vi "Global Read.vi"(0 "VISA #":string, 3 "error in (no error)":errorcluster) -> (4 "Global for this VISA":T1, 5 "VICI Global Array Out":T2, 6 "Pump Array":string[](array[string]), 7 "Busy":bool, 8 "VISA #":string, 9 "Current Pump":string, 10 "error out":errorcluster)   [LabVIEW 2018, in "VICI M6 M50 Party Mode.lvlib" / "VICI Global Library.lvlib"]
uses:
  VICI Global Library.lvlib
  VICI Global Array.ctl
  VICI Global.ctl
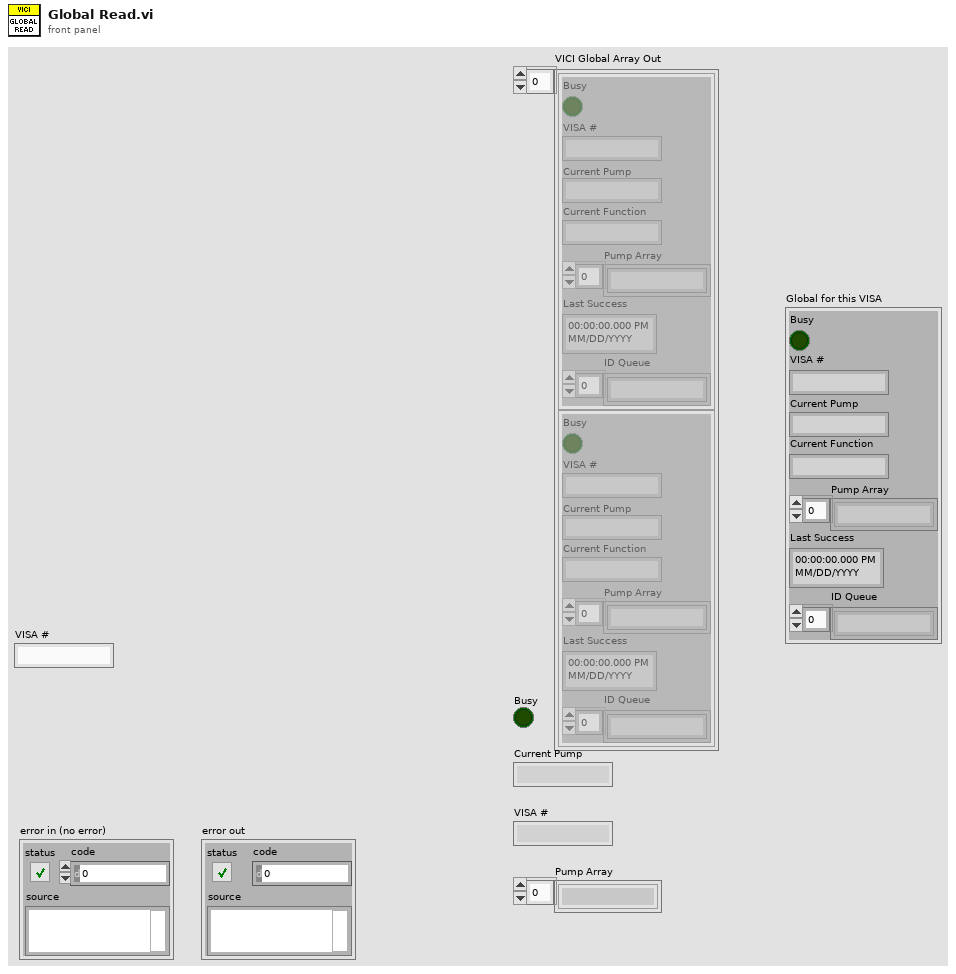
[diagram p1: front panel]
types:
  T1 = typedef "VICI M6 M50 Party Mode.lvlib/VICI Global Library.lvlib/VICI Global.ctl" = cluster{"Busy":bool, "VISA #":string, "Current Pump":string, "Current Function":string, "Pump Array":string[], "Last Success":timestamp, "ID Queue":string[]}
  T2 = typedef "VICI M6 M50 Party Mode.lvlib/VICI Global Library.lvlib/VICI Global Array.ctl" = T1[]
  T3 = cluster{"Busy":bool, "VISA #":string, "Current Pump":string, "Current Function":string, "Pump Array":string[], "Last Success":timestamp, "ID Queue":string[]}[]
  T4 = cluster{"Busy":bool, "VISA #":string, "Current Pump":string, "Current Function":string, "Pump Array":string[], "Last Success":timestamp, "ID Queue":string[]}
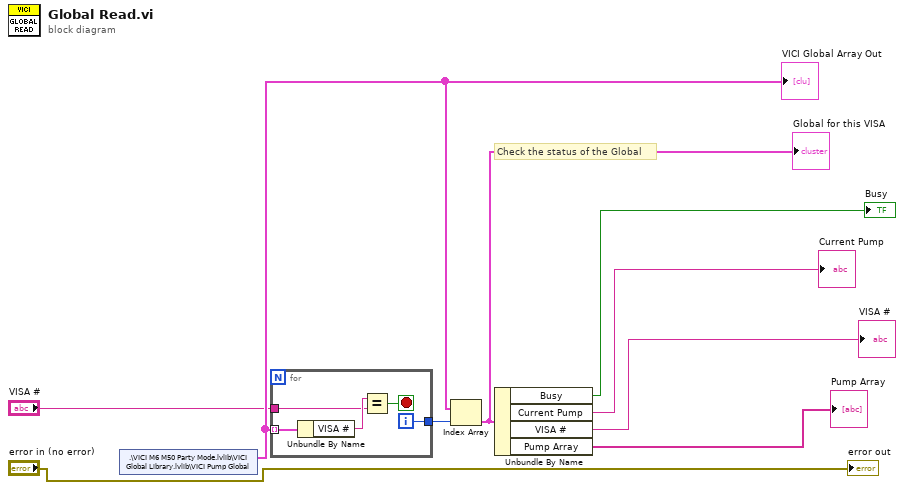
[diagram p0: block diagram]
diagram:
  # "Check the status of the Global"
  n1 = shared-variable ".\\VICI M6 M50 Party Mode.lvlib\\VICI Global Library.lvlib\\VICI Pump Global"() -> (w5:T3)  [unwired: 1 in, 1 out]
  "VICI Global Array Out" <- w5
  n2 = for {
    tunnel: w5 -> [w14] mode=indexing
    tunnel: "VISA #" -> [w12]
    tunnel: [w11] -> w4
    i -> [w11]
    stop <- w10 stop-if-true
    n3 = Unbundle By Name(w14) -> ("VISA #"=w13:string)
    n4 = Equal?(x=w13, y=w12) -> (x = y?=w10:bool)
  }
  n5 = Index Array(array=w5, index=w4) -> (element=w9:T4)
  "Global for this VISA" <- w9
  n6 = Unbundle By Name(w9) -> ("Busy"=→"Busy":bool, "Current Pump"=→"Current Pump":string, "VISA #"=→"VISA #":string, "Pump Array"=→"Pump Array":string[])
  "error out" <- "error in (no error)"
